vi "SendCommand.vi"(10 "Command":string="{\n   \"command_type\":\"LevelZero\",\n   \"command\":\n   {\n      \"LevelZero_command_type\":\"Power Switch\",\n      \"LevelZero_command\":{\"Switch\":\"Flight Computer\",\"Switch State\":\"On\"}\n   }\n}", 11 "Queue In":refnum<queue>) -> (3 "Queue Out":refnum<queue>)   [LabVIEW 2014]
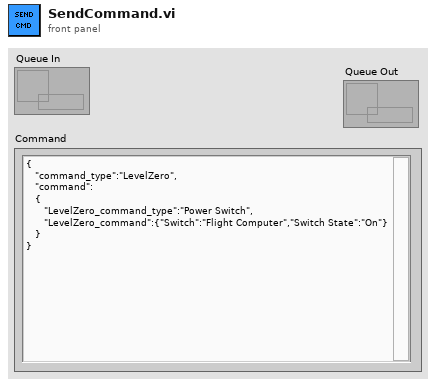
[diagram p1: front panel]
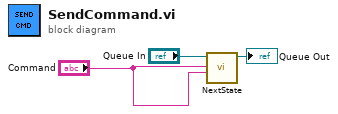
[diagram p0: block diagram]
diagram:
  n1 = call "NextState.vi"("Data"="Command", "State"="Command", "Queue In"="Queue In") -> ("Queue Out"=→"Queue Out":refnum<queue>)  [unwired: 7 in, 1 out]
